vi "数据成组.vi"(0 "数据个数":i32=5) -> (1 "输出数组":i32[](array[numeric]), 2 "数据个数":i32=5)   [LabVIEW 2019]
uses:
  <vilib>/numeric/Random Number (Range) I64.vi
  <vilib>/numeric/sub_Random U32.vi
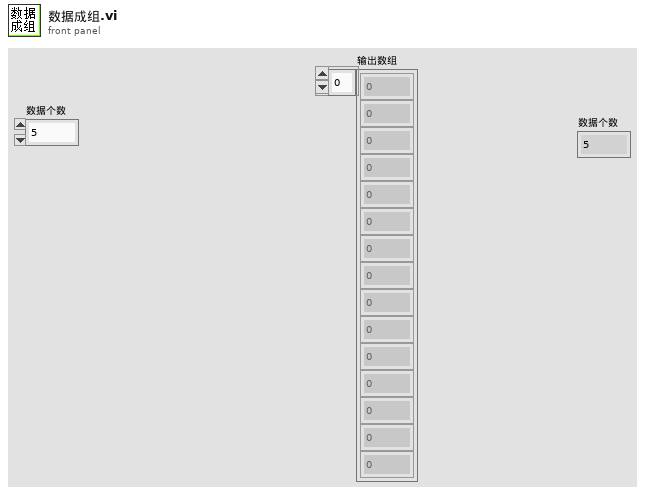
[diagram p1: front panel]
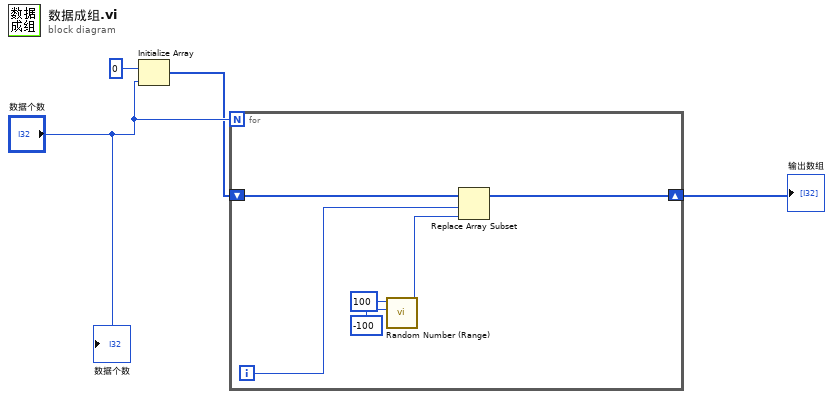
[diagram p0: block diagram]
diagram:
  n1 = Initialize Array(0 ("元素"), "数据个数") -> (w1:i32[])
  n2 = for {
    N: "数据个数" -> [_]
    shift-right: [w9] -> w3
    shift-left: w1 -> [w8]
    i -> [w10]
    n3 = call-poly <vilib>:"Random Number (Range).vi"("lower bound (-100)"=-100 ("lower bound (0)"), "upper bound (100)"=100) -> ("number"=w5:i64)  [unwired: 9 in]
    n4 = Replace Array Subset(array=w8, new element=w5, index=w10) -> (w9:i32[])
  }
  "输出数组" <- w3
  "数据个数" <- "数据个数"
